vi "Handle Execution Mode.vi"(8 "error in (no error)":errorcluster, 10 "Execution Mode":T1, 11 "Execution UI In":refnum<class "Execution UI.lvclass">) -> (0 "error out":errorcluster, 3 "Execution UI Out":refnum<class "Execution UI.lvclass">)   [LabVIEW 2020, in "Execution UI.lvclass"]
uses:
  Execution UI.lvclass
  C:/Users/anton/Documents/GitHub/LUnit/source/Application Framework/Process Classes/Process/Process.lvclass
  Public/Execution Mode.ctl
  Execution UI.lvclass/Execution UI.ctl
  Helper Classes/Buffered Test Finder/Indexing Test Finder.lvclass
  C:/Users/anton/Documents/GitHub/LUnit/source/Framework/Helper Classes/Test Finder/Test Finder.lvclass
  Application Framework/Process Classes/Process/Process.lvclass/Process.ctl
  Helper Classes/Buffered Test Finder/Indexing Test Finder.lvclass/Indexing Test Finder.ctl
  Helper Classes/Test Finder/Test Finder.lvclass
  Application Framework/Process Classes/Process/Protected/Messaging/Enqueue Message.vi
  Icon Decorator/Icon Decorator.lvclass
  Helper Classes/Test Finder/Public/SubVIs/Register For Test Cases Found Event.vi
  Application Framework/Process Classes/Process/Process.lvclass
  C:/Users/anton/Documents/GitHub/LUnit/source/Framework/Execution UI/Execution UI.lvclass
  C:/Users/anton/Documents/GitHub/LUnit/source/Framework/Helper Classes/Buffered Test Finder/Indexing Test Finder.lvclass
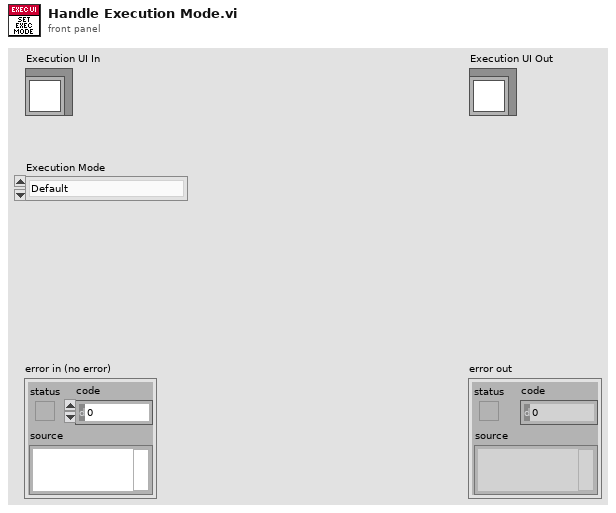
[diagram p1: front panel]
types:
  T1 = typedef "Execution UI.lvclass/Execution Mode.ctl" = enum16{"Default", "Run Tests In Project", "Run Test Case"}
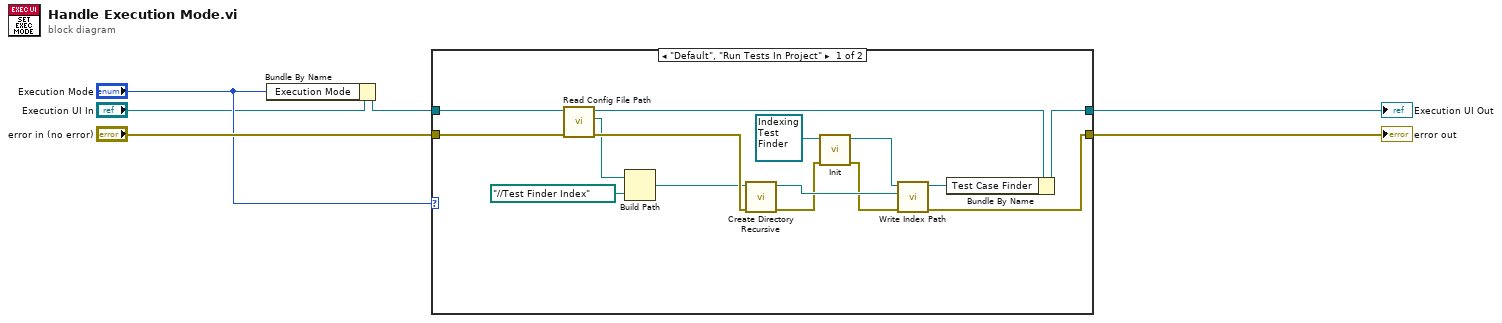
[diagram p0: block diagram]
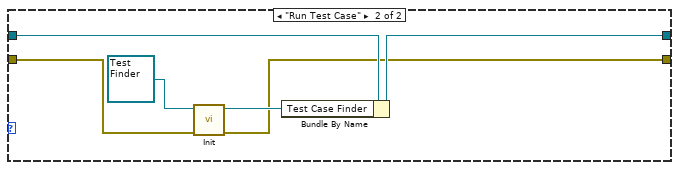
[diagram p2: hidden frame]
diagram:
  n1 = Bundle By Name(cluster="Execution UI In", "Execution Mode"="Execution Mode") -> (w3:refnum<class "Execution UI.lvclass">)
  n2 = case shown="\"Default\", \"Run Tests In Project\"" "Execution Mode" {
    tunnel: [w11 w27] -> w5
    tunnel: w3 -> [w16 w26]
    tunnel: [w13 w23] -> w4
    tunnel: "error in (no error)" -> [w15 w22]
    frame "Default", "Run Tests In Project" {
      n3 = call "Read Config File Path.vi"("error in (no error)"=w15, "Process In"=w16) -> ("error out"=w20:errorcluster, "Config File Path"=w19:path, "Process Out"=w21:refnum<class "Execution UI.lvclass">)  [unwired: 7 in]
      n4 = Build Path(base path=w19, name or relative path=path "../../Test Finder Index") -> (appended path=w17:path)
      n5 = call <vilib>:"Create Directory Recursive.vi"("error in (no error)"=w20, "directory"=w17) -> ("error out"=w8:errorcluster, "directory copy"=w14:path)  [unwired: 3 in, 1 out]
      n6 = call-dynamic "Init.vi"("error in (no error)"=w8, "Test Finder in"=refnum<class "Indexing Test Finder.lvclass"> refnum ("Indexing Test Finder.lvclass")) -> ("error out"=w7:errorcluster, "Test Finder out"=w9:refnum<class "Indexing Test Finder.lvclass">)  [unwired: 8 in]
      n7 = call "Write Index Path.vi"("error in (no error)"=w7, "Index Folder Path"=w14, "Indexing Test Finder in"=w9) -> ("error out"=w13:errorcluster, "Indexing Test Finder out"=w10:refnum<class "Indexing Test Finder.lvclass">)  [unwired: 7 in]
      n8 = Bundle By Name(cluster=w21, "Test Case Finder"=w10) -> (w11:refnum<class "Execution UI.lvclass">)
    }
    frame "Run Test Case" {
      n9 = call-dynamic "Init.vi"("error in (no error)"=w22, "Test Finder in"=refnum<class "Test Finder.lvclass"> refnum ("Test Finder.lvclass")) -> ("error out"=w23:errorcluster, "Test Finder out"=w24:refnum<class "Test Finder.lvclass">)  [unwired: 8 in]
      n10 = Bundle By Name(cluster=w26, "Test Case Finder"=w24) -> (w27:refnum<class "Execution UI.lvclass">)
    }
  }
  "error out" <- w4
  "Execution UI Out" <- w5
